vi "op_x2_GetIDs.vi"(1 "ENA1":bool caption="Connection 1 enable", 2 "IP address 1":string="172.16.14.22", 5 "ENA2":bool caption="Connection 2 enable", 6 "IP address 2":string="172.16.14.23") -> (16 "summary IDs":string, 20 "All ID list 1":u32[](array[numeric]) format="%.0x", 21 "Layer ID list 1 (ordered)":u32[](array[numeric]) format="%.0x", 22 "Chip ID list 1":u32[](array[numeric]) format="%.0x", 24 "All ID list 2":u32[](array[numeric]) format="%.0x", 25 "Layer ID list 2 (ordered)":u32[](array[numeric]) format="%.0x", 26 "Chip ID list 2":u32[](array[numeric]) format="%.0x", 27 "error out":errorcluster)   [LabVIEW 2015, in "VIPM2.lvlib"]
doc: "Operation: <b>GetID</b> from 2 FPGAs simultaneously.\nFa dues crides a <b>op_GetIDs.vi</b> amb reentrança.\nConstrueix el summary IDs conjunt per a la app."
uses:
  VIPM2.lvlib
panel:
  # "Operation: GetID from 2 FPGAs simultaneously"
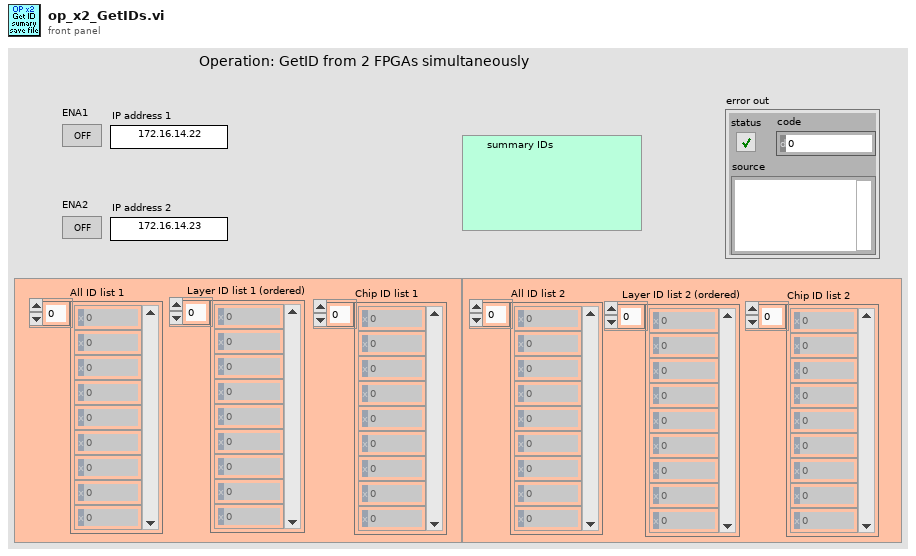
[diagram p1: front panel]
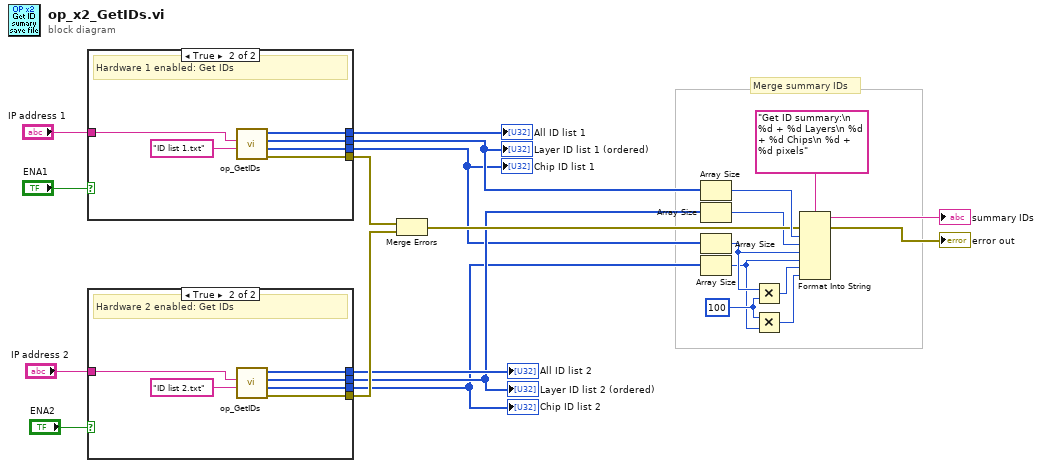
[diagram p0: block diagram]
diagram:
  w2 = 100 ("y")
  # "Merge summary IDs"
  n1 = case shown="True" "ENA1" {
    tunnel: "IP address 1" -> [_ w28]
    tunnel: [_ w27] -> w18
    tunnel: [_ w26] -> w8
    tunnel: [_ w25] -> w13
    tunnel: [_ w24] -> w17
    frame False {
      # "Hardware 1 not enabled"
    }
    frame True {
      # "Hardware 1 enabled: Get IDs"
      n2 = call "op_GetIDs.vi"("list ID file name"="ID list 1.txt", "IP address"=w28) -> ("error out"=w27:errorcluster, "Chip ID list"=w26:u32[], "Layer ID list (ordered)"=w25:u32[], "All ID list"=w24:u32[])  [unwired: 5 in, 1 out]
    }
  }
  "All ID list 1" <- w17
  "Layer ID list 1 (ordered)" <- w13
  "Chip ID list 1" <- w8
  n3 = case shown="True" "ENA2" {
    tunnel: "IP address 2" -> [_ w34]
    tunnel: [_ w33] -> w19
    tunnel: [_ w32] -> w6
    tunnel: [_ w31] -> w9
    tunnel: [_ w30] -> w16
    frame False {
      # "Hardware 2 not enabled"
    }
    frame True {
      # "Hardware 2 enabled: Get IDs"
      n4 = call "op_GetIDs.vi"("list ID file name"="ID list 2.txt", "IP address"=w34) -> ("error out"=w33:errorcluster, "Chip ID list"=w32:u32[], "Layer ID list (ordered)"=w31:u32[], "All ID list"=w30:u32[])  [unwired: 5 in, 1 out]
    }
  }
  "All ID list 2" <- w16
  "Layer ID list 2 (ordered)" <- w9
  "Chip ID list 2" <- w6
  n5 = Merge Errors "Merge Errors"(w18, w19) -> (w11:errorcluster)
  n6 = Array Size(array=w13) -> (size(s)=w12:i32)
  n7 = Array Size(array=w9) -> (size(s)=w7:i32)
  n8 = Array Size(array=w8) -> (size(s)=w5:i32)
  n9 = Array Size(array=w6) -> (size(s)=w1:i32)
  n10 = Multiply(x=w5, y=w2) -> (x*y=w4:i32)
  n11 = Multiply(x=w2, y=w1) -> (x*y=w3:i32)
  n12 = Format Into String "Format Into String"(format string="Get ID summary:\n %d + %d Layers\n %d + %d Chips\n %d + %d pixels", error in=w11, w12, w7, w5, w1, w4, w3) -> (resulting string=→"summary IDs":string, error out=→"error out":errorcluster)  [unwired: 1 in]
